vi "Save Offsets.vi"(8 "error in (no error)":errorcluster) -> (0 "error out":errorcluster)   [LabVIEW 2009]
uses:
  Apps/App Parameters Actions.ctl
  Logging/LogFileType.ctl
  Data Access Objects/Metadata/DAO Actions.ctl
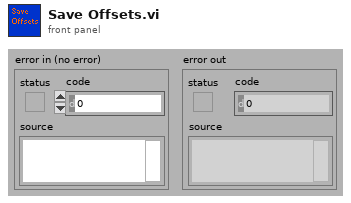
[diagram p1: front panel]
types:
  T1 = typedef "DAO Actions.ctl" = enum16{"Init", "Get", "Set"}
  T2 = typedef "LogFileType.ctl" = enum16{"Continuous", "Step", "Volts", "Offsets", "DLL  Errors", "Snapshot", "Commands", "StiffnessUpdates", "End List"}
  T3 = typedef "App Parameters Actions.ctl" = enum16{"Init", "Get", "Set"}
  T4 = typedef "Dataset Transaction Id.ctl" = cluster{"Dataset Source":T5, "Dataset Type":T6, "Hold":T7, "Volts":T7, "Tag":string}
  T5 = typedef "Dataset Source.ctl" = enum16{"LBCB 1", "LBCB 2", "Combined", "External Sensors"}
  T6 = typedef "Dataset Type.ctl" = enum16{"LVDT", "Load Cell", "Actuator Command", "Servo Error", "Displacement Command", "Displacement", "Force"}
  T7 = typedef "Yes No Button.ctl" = bool
  T8 = typedef "App Parameters.ctl" = cluster{"Monitor Loop":T9, "Ramp Time":T9, "Log Loop":T9, "TCP to DAQ":T9, "Logging Directory":path, "Log File Size (MBytes)":i64, "Volt Logging Loop":T9, "2 LBCB Archiving Mode":bool}
  T9 = typedef "Timing Parameters.ctl" = cluster{"Interval":dbl, "Rate ":dbl}
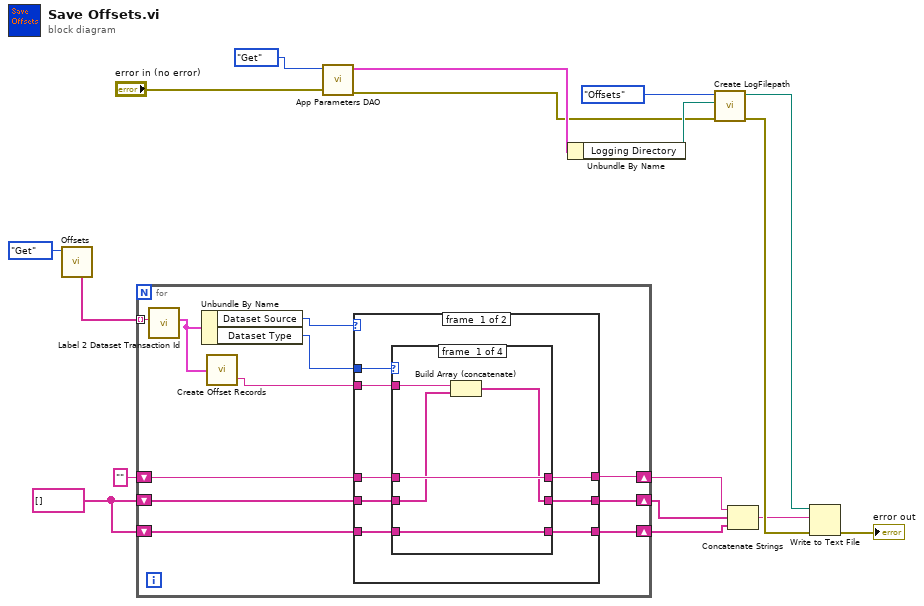
[diagram p0: block diagram]
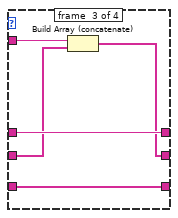
[diagram p3: hidden frame]
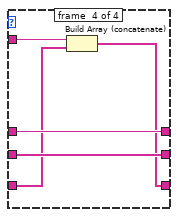
[diagram p4: hidden frame]
diagram:
  w1 = string[] []
  n1 = call "Offsets.vi"("DAO Actions"=DAO_Actions."Get") -> ("Labels"=w7:string[])  [unwired: 8 in, 2 out]
  n2 = for {
    tunnel: w7 -> [w28] mode=indexing
    shift-right: [w23] -> w6
    shift-left: w1 -> [w19]
    shift-right: [w22] -> w5
    shift-left: w1 -> [w20]
    shift-right: [w21] -> w4
    shift-left: "" ("record") -> [w18]
    n3 = call "Label 2 Dataset Transaction Id.vi"("Label"=w28) -> ("Dataset Trans Id"=w27:T4)  [unwired: 10 in]
    n4 = Unbundle By Name(w27) -> ("Dataset Source"=w26:T5, "Dataset Type"=w25:T6)
    n5 = call "Create Offset Records.vi"("Dataset Trans Id"=w27) -> ("record"=w24:string)  [unwired: 1 in]
    n6 = case shown="\"External Sensors\"" w26 {
      tunnel: w25 -> [w36 _]
      tunnel: w24 -> [w35 w57]
      tunnel: [w34 w55] -> w23
      tunnel: [w33 w56] -> w22
      tunnel: [w31 w57] -> w21
      tunnel: w20 -> [w29 w56]
      tunnel: w19 -> [w30 w55]
      tunnel: w18 -> [w32 _]
      frame #0 {
        n7 = case shown="\"LVDT\"" w36 {
          tunnel: w35 -> [w39 _ w47 w52]
          tunnel: [w40 w42 w48 w50] -> w34
          tunnel: [w37 w43 w45 w53] -> w33
          tunnel: w32 -> [w41 w44 w49 w54]
          tunnel: [w41 w44 w49 w54] -> w31
          tunnel: w30 -> [w40 w42 w48 w51]
          tunnel: w29 -> [w38 w43 w46 w53]
          frame #0 {
            n8 = Build Array (concatenate)(w39, w38) -> (w37:string[])
          }
          frame #1 {
          }
          frame #2 {
            n9 = Build Array (concatenate)(w47, w46) -> (w45:string[])
          }
          frame #3 {
            n10 = Build Array (concatenate)(w52, w51) -> (w50:string[])
          }
        }
      }
      frame #1 {
      }
    }
  }
  n11 = call "App Parameters DAO.vi"("error in (no error)"="error in (no error)", "Actions"=App_Parameters_Actions."Get" ("App Parameter Actions")) -> ("error out"=w13:errorcluster, "Application Timing and Logging Out"=w16:T8)  [unwired: 2 in, 6 out]
  n12 = Unbundle By Name(w16) -> ("Logging Directory"=w15:path)
  n13 = call "Create LogFilepath.vi"("error in (no error)"=w13, "Log Directory"=w15, "LogFile Type"=LogFileType."Offsets") -> ("error out"=w9:errorcluster, "Logfile Path"=w12:path)  [unwired: 7 out]
  n14 = Concatenate Strings(w4, w5, w6) -> (w3:string)
  n15 = Write to Text File(file (use dialog)=w12, text=w3, error in=w9) -> (error out=→"error out":errorcluster)  [unwired: 3 out]
